vi "Part 1.vi"(11 "Input":string) -> (3 "Output":i64)   [LabVIEW 2021]
uses:
  <vilib>/regexp/Match Regular Expression.xnode
  <userlib>/_OpenG.lib/string/string.llb/Convert EOLs (String)__ogtk.vi
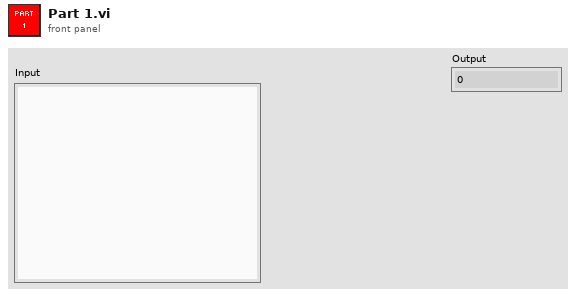
[diagram p1: front panel]
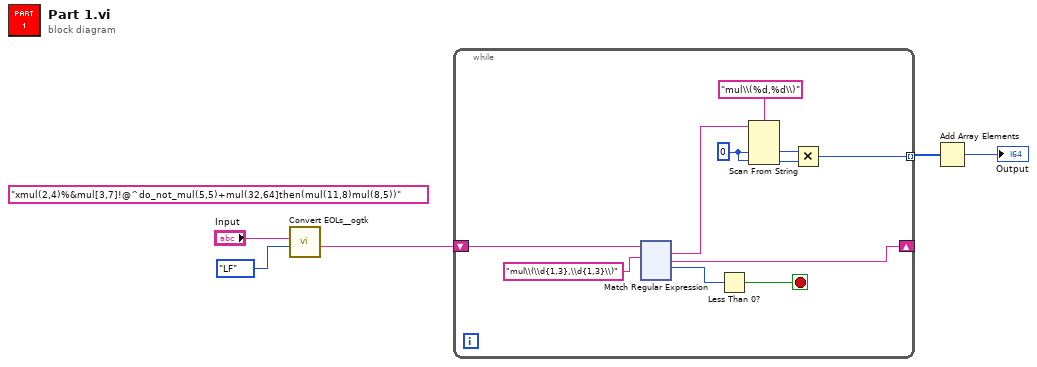
[diagram p0: block diagram]
diagram:
  (unwired) "xmul(2,4)%&mul[3,7]!@^do_not_mul(5,5)+mul(32,64]then(mul(11,8)mul(8,5))"
  n1 = call-poly <userlib>:"Convert EOLs__ogtk.vi"("Convert to:"=enum16{"CR", "LF", "CRLF"}."LF", "String in"="Input") -> ("String out"=w4:string)  [unwired: 9 in]
  n2 = while {
    shift-right: [w15] -> _
    shift-left: w4 -> [w16]
    tunnel: [w7] -> w3 mode=indexing
    stop <- w13 stop-if-true
    w6 = i64 0
    n3 = xnode "Match Regular Expression"("input string"=w16, "regular expression"="mul\\(\\d{1,3},\\d{1,3}\\)") -> ("whole match"=w11:string, "after match"=w15:string, "offset past match"=w14:i32)  [unwired: 4 in, 2 out]
    n4 = Less Than 0?(x=w14) -> (x < 0?=w13:bool)
    n5 = Scan From String(format string="mul\\(%d,%d\\)", input string=w11, default 1=w6, default 2=w6) -> (output 1=w8:i64, output 2=w9:i64)  [unwired: 2 in, 3 out]
    n6 = Multiply(x=w8, y=w9) -> (x*y=w7:i64)
  }
  n7 = Add Array Elements(numeric array=w3) -> (sum=→"Output":i64)
